vi "Test analog.vi"() -> ()   [LabVIEW 2017]
uses:
  <vilib>/Instr/_visa.llb/VISA Configure Serial Port (Instr).vi
panel:
  out "concatenated string":string
  in  "VISA resource name":refnum<visa-resource-name>
  in  "stop":bool
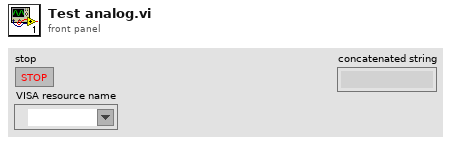
[diagram p1: front panel]
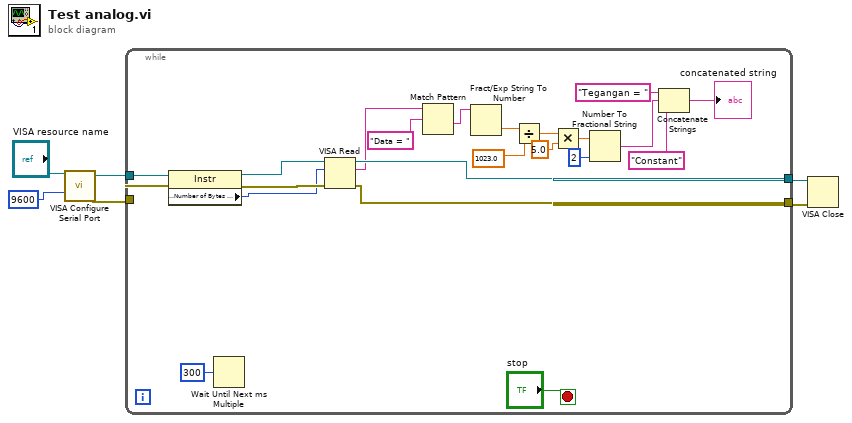
[diagram p0: block diagram]
diagram:
  n1 = call-poly "VISA Configure Serial Port"("VISA resource name"="VISA resource name", "baud rate (9600)"=u32 9600 ("byte count")) -> ("VISA resource name out"=w5:refnum<visa-resource-name>, "error out"=w4:errorcluster)  [unwired: 12 in]
  n2 = while {
    tunnel: [w28] -> w6
    tunnel: w5 -> [w24]
    tunnel: w4 -> [w23]
    tunnel: [w22] -> w3
    stop <- "stop" stop-if-true
    n3 = property class="Instr"(reference=w24, error in=w23) -> (reference out=w25:refnum<visa-resource-name>, error out=w27:errorcluster, "Serial Settings:Number of Bytes at Serial Port"=w26:u32)
    n4 = Wait Until Next ms Multiple(millisecond multiple=u32 300) -> ()  [unwired: 1 out]
    n5 = VISA Read(VISA resource name=w25, byte count=w26, error in (no error)=w27) -> (VISA resource name out=w22:refnum<visa-resource-name>, read buffer=w19:string, error out=w28:errorcluster)  [unwired: 1 out]
    n6 = Match Pattern(string=w19, regular expression="Data = ") -> (after substring=w17:string)  [unwired: 1 in, 3 out]
    n7 = Fract/Exp String To Number(string=w17) -> (number=w16:dbl)  [unwired: 3 in, 1 out]
    n8 = Divide(x=w16, y=1023.0) -> (x/y=w14:dbl)
    n9 = Multiply(x=w14, y=5.0) -> (x*y=w12:dbl)
    n10 = Number To Fractional String(number=w12, width (-)=i16 2) -> (F-format string=w9:string)  [unwired: 2 in]
    n11 = Concatenate Strings("Tegangan = " ("string"), w9, "Constant" ("string")) -> (→"concatenated string":string)
  }
  n12 = VISA Close(VISA resource name=w3, error in (no error)=w6) -> ()  [unwired: 1 out]
